vi "GetDeviceFromSignal.vi"(8 "Error in":errorcluster, 10 "Signal":refnum<k24>, 11 "DevicesAndSignals":T1) -> (0 "Error out":errorcluster, 2 "Device":refnum<k24>, 3 "DevicesAndSignals":T1)   [LabVIEW 2016]
doc: "Finds the device to which the given signal belongs.\n\nSignal: Signal to check to which device it belongs\nDevice: The device to which the signal belongs"
uses:
  C:/Users/CL/Desktop/ZcDAQprj0811/ZcDAQprj/Modules/DAQ-Device/Hardware Drivers/QX/HBM LabVIEW Driver/DLLs/Hbm.Api.Common.dll
  DLLs/Hbm.Api.Common.dll
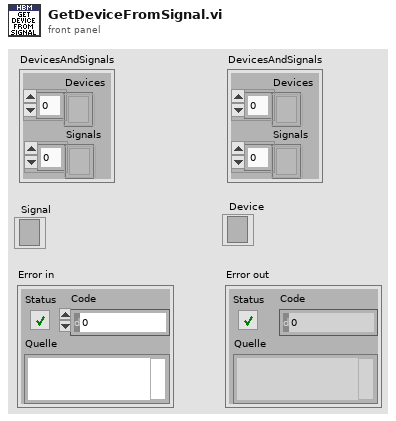
[diagram p1: front panel]
types:
  T1 = cluster{"Devices":refnum<k24>[], "Signals":refnum<k24>[]}
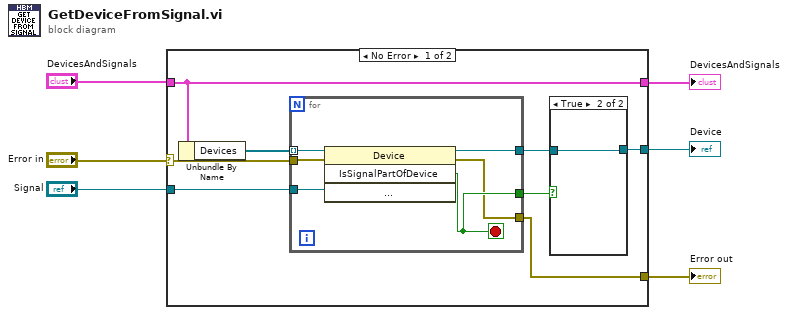
[diagram p0: block diagram]
diagram:
  n1 = case shown="No Error" "Error in" {
    selector: "Error in" -> [w8 w23]
    tunnel: [w7 w23] -> w6
    tunnel: [w14 w22] -> w3
    tunnel: "DevicesAndSignals" -> [w14 w22]
    tunnel: [w12 _] -> w2
    tunnel: "Signal" -> [w11 _]
    frame No Error {
      n2 = Unbundle By Name(w14) -> ("Devices"=w13:refnum<k24>[])
      n3 = for {
        tunnel: w13 -> [w21] mode=indexing
        tunnel: w11 -> [w20]
        tunnel: [w19] -> w10
        tunnel: [w18] -> w9
        tunnel: w8 -> [w17]
        tunnel: [w16] -> w7
        stop <- w19 stop-if-true
        n4 = invoke on="Methodenknoten" class="Device" method="IsSignalPartOfDevice"(reference=w21, error in=w17, "signalToCheck"=w20) -> (reference out=w18:refnum<k24>, error out=w16:errorcluster, "IsSignalPartOfDevice"=w19:bool)  [unwired: 1 in, 1 out]
      }
      n5 = case shown="True" w10 {
        tunnel: [_ w15] -> w12
        tunnel: w9 -> [_ w15]
        frame False {
        }
        frame True {
        }
      }
    }
    frame Error {
    }
  }
  "Error out" <- w6
  "DevicesAndSignals" <- w3
  "Device" <- w2
